vi "XYZ_translation_doubleside.vi"() -> ()   [LabVIEW 2021]
uses:
  C:/Program Files (x86)/Control/SC3U.dll
  Program Files (x86)/Control/SC3U.dll
  <instrlib>/Xbox-One-Controller/Private/Type Defs/Indicators/Controller.ctl
  <instrlib>/Xbox-One-Controller/Private/Type Defs/Indicators/A.ctl
  <instrlib>/Xbox-One-Controller/Private/Type Defs/Indicators/B.ctl
  <instrlib>/Xbox-One-Controller/Private/Type Defs/Indicators/X.ctl
  <instrlib>/Xbox-One-Controller/Private/Type Defs/Indicators/Y.ctl
  <instrlib>/Xbox-One-Controller/Private/Type Defs/Indicators/Left Bumper.ctl
  <instrlib>/Xbox-One-Controller/Private/Type Defs/Indicators/Right Bumper.ctl
  <instrlib>/Xbox-One-Controller/Private/Type Defs/Indicators/View.ctl
  <instrlib>/Xbox-One-Controller/Private/Type Defs/Indicators/Menu.ctl
  <instrlib>/Xbox-One-Controller/Private/Type Defs/Indicators/Thumbstick_Analog.ctl
  <instrlib>/Xbox-One-Controller/Private/Type Defs/Indicators/Slider.ctl
  <instrlib>/Xbox-One-Controller/Private/Type Defs/Indicators/DPad.ctl
  <vilib>/Platform/TimedLoop/XDataNode/timing_clust.ctl
  <vilib>/Platform/TimedLoop/XDataNode/nitl_modes.ctl
  <vilib>/Platform/TimedLoop/XDataNode/wakeup.ctl
  <instrlib>/Xbox-One-Controller/Public/Open First Controller.vi
  <vilib>/Platform/TimedLoop/XDataNode/XDataNode.xnode
  <vilib>/Platform/TimedLoop/XDataNode/XDNodeRunTimeDep.lvlib
  <instrlib>/Xbox-One-Controller/LMH-Xbox-One-Controller.lvlib
panel:
  in  "Front Panel Window:Is Frontmost":bool
  in  "Displace Stamp Y":i64=1
  in  "Displace Stamp X":i64=1
  in  "Displace Sample R":i64=1
  out "Pos Stamp Y":dbl
  out "Pos Stamp X":dbl
  out "Pos Sample R":dbl
  in  "Displace Divided by 5":bool caption="Boolean 2"
  in  "Displace Multip by 5":bool caption="Boolean"
  out "Pos Sample X":dbl
  out "Pos Sample Z":dbl
  in  "Displace Sample Z":i64=1
  out "Pos Sample Y":dbl
  in  "Displace Sample Y":i64
  in  "Stop Button":bool
  out "Controller":T1={"A Button"=FALSE, "B Button"=FALSE, "X Button"=FALSE, "Y Button"=FALSE, "Left Bumper"=FALSE, "Right Bumper"=FALSE, "View Button"=FALSE, "Menu Button"=FALSE, "Left Stick"={[], []}, "Right Stick"={[], []}, "Trigger"=0, "D-Pad"=5} {"Trigger" scale=32767.0..-32768.0}
  in  "SC3U":refnum<k24>(container)
  in  "Com Close":bool
  in  "Displace Sample X":i64
  out "ConnectStatus":bool
  out "ComUsing":i16
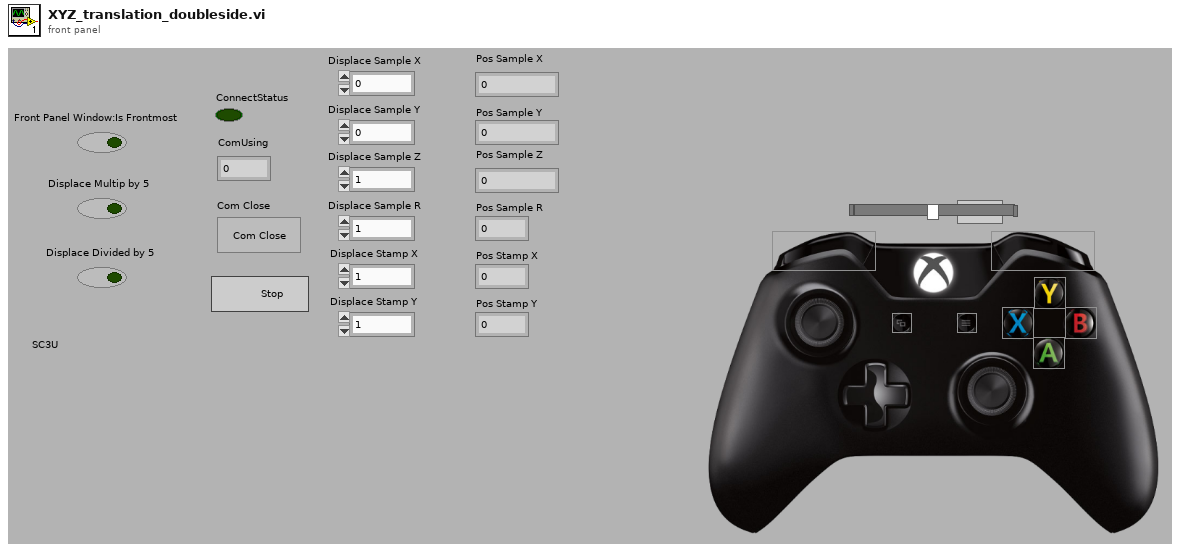
[diagram p1: front panel]
types:
  T1 = typedef "LMH-Xbox-One-Controller.lvlib/Controller.ctl" = cluster{"A Button":T2, "B Button":T3, "X Button":T4, "Y Button":T5, "Left Bumper":T6, "Right Bumper":T7, "View Button":T8, "Menu Button":T9, "Left Stick":T10, "Right Stick":T10, "Trigger":T11, "D-Pad":T12}
  T2 = typedef "LMH-Xbox-One-Controller.lvlib/A.ctl" = bool
  T3 = typedef "LMH-Xbox-One-Controller.lvlib/B.ctl" = bool
  T4 = typedef "LMH-Xbox-One-Controller.lvlib/X.ctl" = bool
  T5 = typedef "LMH-Xbox-One-Controller.lvlib/Y.ctl" = bool
  T6 = typedef "LMH-Xbox-One-Controller.lvlib/Left Bumper.ctl" = bool
  T7 = typedef "LMH-Xbox-One-Controller.lvlib/Right Bumper.ctl" = bool
  T8 = typedef "LMH-Xbox-One-Controller.lvlib/View.ctl" = bool
  T9 = typedef "LMH-Xbox-One-Controller.lvlib/Menu.ctl" = bool
  T10 = typedef "LMH-Xbox-One-Controller.lvlib/Thumbstick_Analog.ctl" = cluster{i32[], i32[]}
  T11 = typedef "LMH-Xbox-One-Controller.lvlib/Slider.ctl" = i32
  T12 = typedef "LMH-Xbox-One-Controller.lvlib/DPad.ctl" = u16
  T13 = typedef "XDNodeRunTimeDep.lvlib/timing_clust.ctl" = cluster{"Expected End [f-1]":u64, "Actual End [f-1]":u64, "Finished Late? [f-1]":bool, "Expected End [i-1]":u64, "Actual End [i-1]":u64, "Finished Late? [i-1]":bool, "Expected Start [i]":u64, "Actual Start [i]":u64, "Expected Start [f]":u64, "Actual Start [f]":u64, "Source Name":string, "Structure Name":string, "Period":i64, "Deadline":i64, "Offset":i64, "Start":i64, "Priority":i32, "Timeout":i32, "Mode":T14, "Wakeup Reason":T15, "Error":errorcluster, "Source Type":string, "Secondary Source Type":string, "Global End Time":u64, "Global Start Time":u64, "Frame Duration":u64, "Iteration Duration":u64, "Assigned CPU":i32, "I/O Scan Engine Mode":u32}
  T14 = typedef "XDNodeRunTimeDep.lvlib/nitl_modes.ctl" = enum32{"No Change", "Process missed periods, maintain original phase", "Discard missed periods, maintain original phase", "Process missed periods, ignore original phase", "Discard missed periods, ignore original phase"}
  T15 = typedef "XDNodeRunTimeDep.lvlib/wakeup.ctl" = enum32{"Normal", "Aborted", "Asynchronous wakeup", "Timing source error", "Timed loop error", "Timeout"}
  T16 = typedef "LMH-Xbox-One-Controller.lvlib/Xbox One Controller Ref.ctl" = cluster{"Controller Ref":refnum<k1>, "Event Refnum":refnum<event-registration>, "Worker Ref":refnum<vi>}
  T17 = typedef "LMH-Xbox-One-Controller.lvlib/All Axis Data.ctl" = cluster{"Left Stick":cluster{"X Axis":i32, "Y Axis":i32}, "Right Stick":cluster{"X Axis":i32, "Y Axis":i32}, "Triggers":i32, "D-Pad":T18}
  T18 = typedef "LMH-Xbox-One-Controller.lvlib/DPad Enum.ctl" = enum16{"Idle", "Up", "Up / Right", "Right", "Down / Right", "Down", "Down / Left", "Left", "Up / Left"}
  T19 = typedef "LMH-Xbox-One-Controller.lvlib/All Buttons Visual.ctl" = cluster{"A":T2, "B":T3, "X":T4, "Y":T5, "Left Bumper":T6, "Right Bumper":T7, "View Button":T8, "Menu Button":T9, "Left Stick":T20, "Right Stick":T20}
  T20 = typedef "LMH-Xbox-One-Controller.lvlib/Thumbstick.ctl" = bool
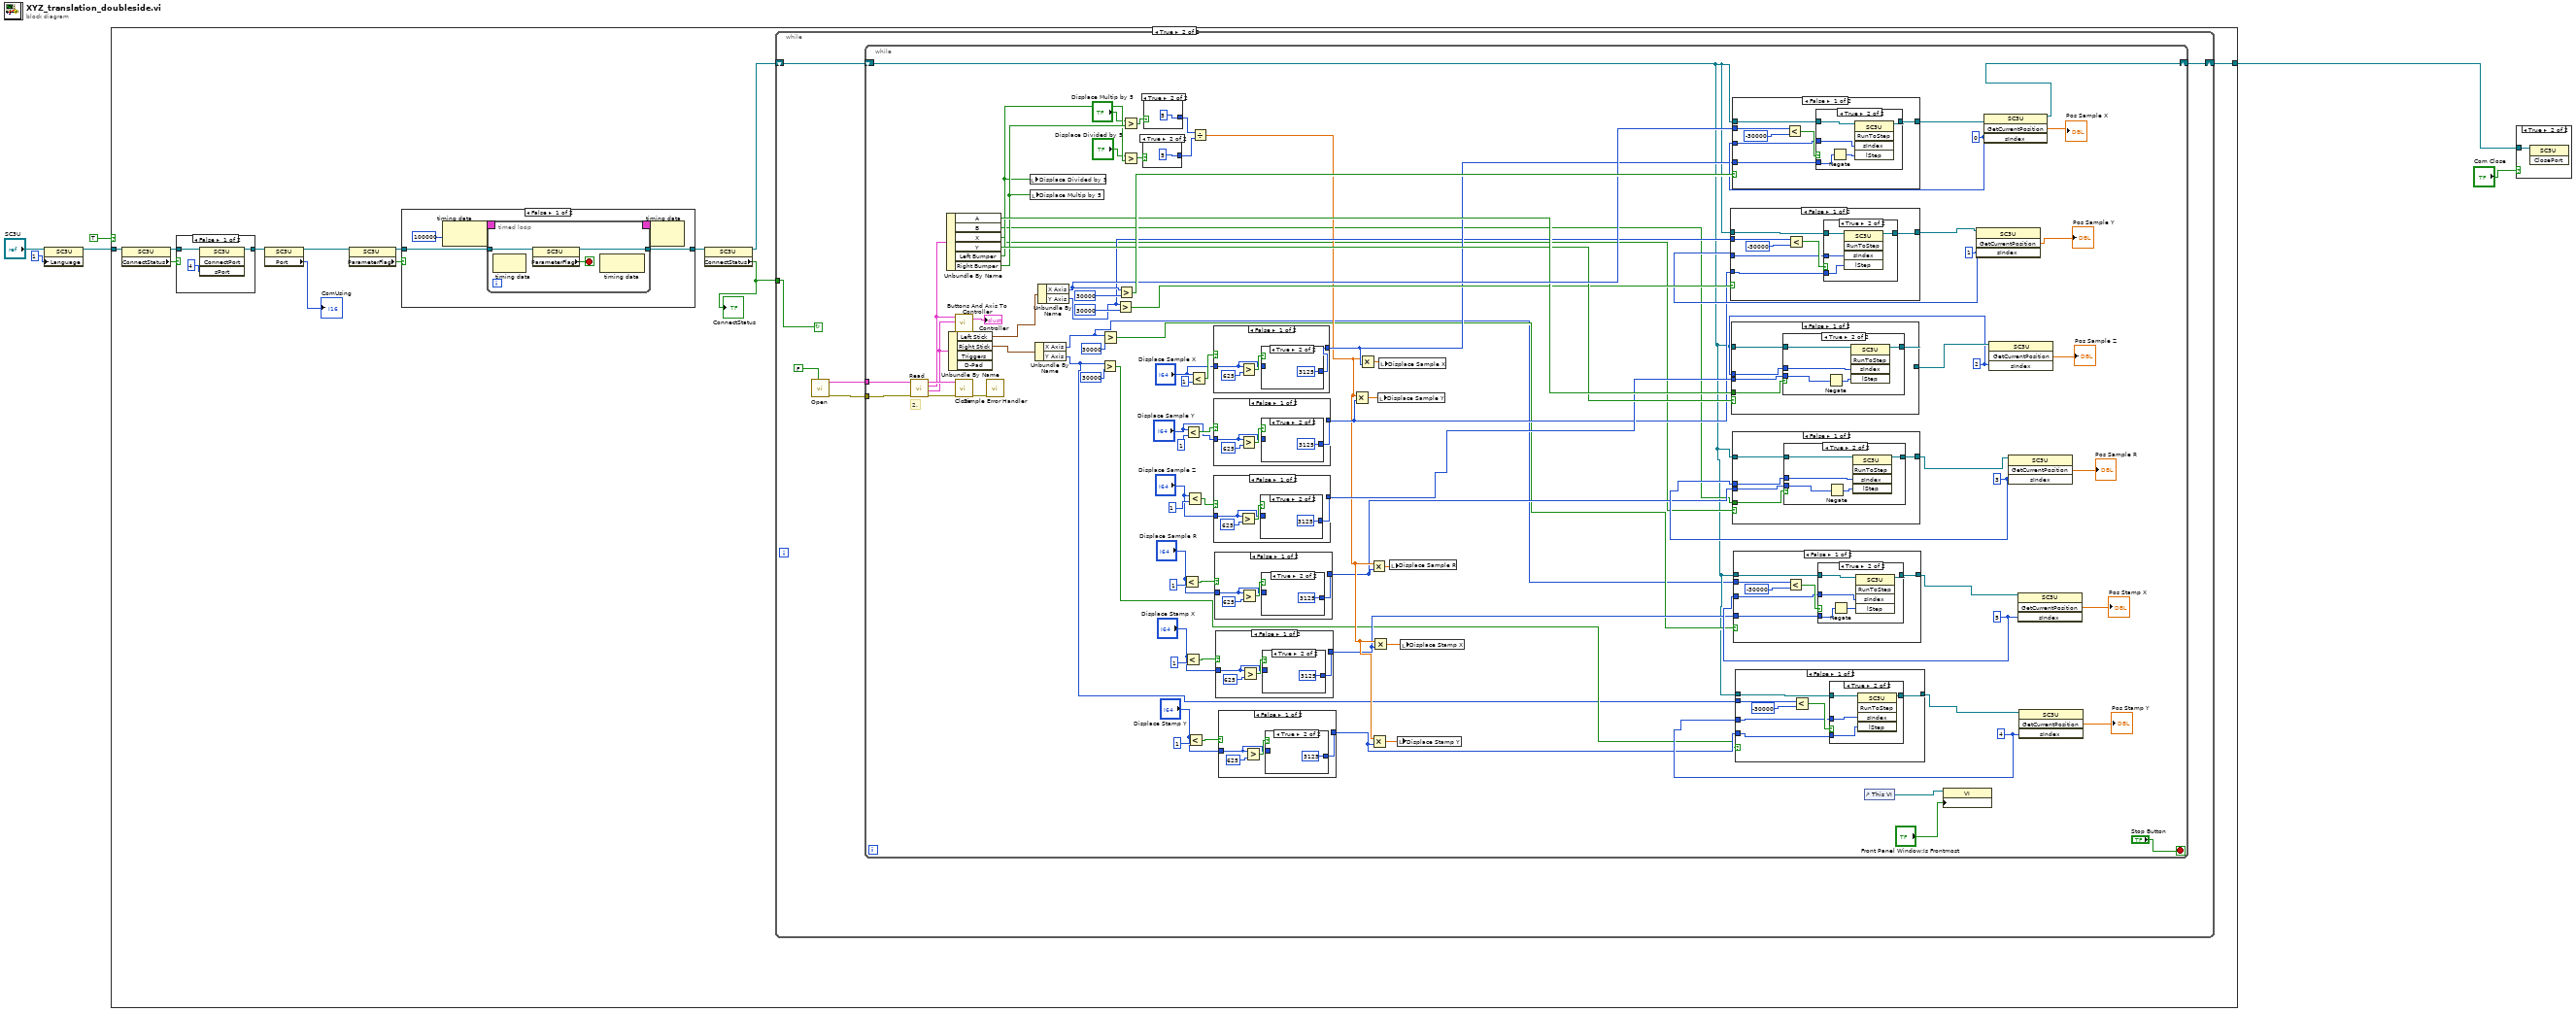
[diagram p0: block diagram]
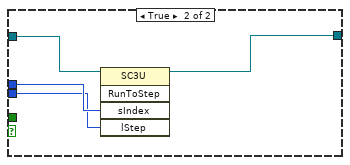
[diagram p5: hidden frame]
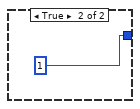
[diagram p7: hidden frame]
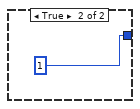
[diagram p9: hidden frame]
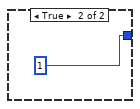
[diagram p11: hidden frame]
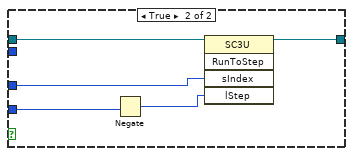
[diagram p13: hidden frame]
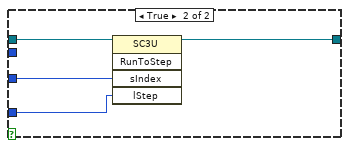
[diagram p15: hidden frame]
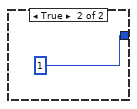
[diagram p17: hidden frame]
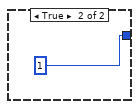
[diagram p19: hidden frame]
diagram:
  n1 = property class="SC3U"(reference="SC3U", "Language"=i16 1 ("intLanguage")) -> (reference out=w1:refnum<k24>)  [unwired: 1 in, 1 out]
  n2 = case shown="True" TRUE {
    tunnel: [_ w8] -> w2
    tunnel: w1 -> [_ w17]
    frame False {
    }
    frame True {
      n3 = property class="SC3U"(reference=w17) -> (reference out=w16:refnum<k24>, "ConnectStatus"=w15:bool)  [unwired: 1 in, 1 out]
      n4 = case shown="False" w15 {
        tunnel: w16 -> [w273 w274]
        tunnel: [w272 w274] -> w14
        frame False {
          n5 = invoke class="SC3U" method="ConnectPort"(reference=w273, "sPort"=i16 4 ("ComUsing")) -> (reference out=w272:refnum<k24>)  [unwired: 2 in, 3 out]
        }
        frame True {
        }
      }
      n6 = property class="SC3U"(reference=w14) -> (reference out=w12:refnum<k24>, "Port"=→"ComUsing":i16)  [unwired: 1 in, 1 out]
      n7 = property class="SC3U"(reference=w12) -> (reference out=w11:refnum<k24>, "ParameterFlag"=w10:bool)  [unwired: 1 in, 1 out]
      n8 = case shown="False" w10 {
        tunnel: w11 -> [w257 w270]
        tunnel: [w256 w270] -> w18
        frame False {
          n9 = node-c288(i64 100000 ("周期")) -> (w260:T13)
          n10 = timed-loop {
            timing: w260 -> [_]
            timing-out: [_] -> w259
            tunnel: w257 -> [w263]
            tunnel: [w262] -> w256
            stop <- w261 stop-if-true
            n11 = node-c288() -> ()  [unwired: 1 in, 1 out]
            n12 = property class="SC3U"(reference=w263) -> (reference out=w262:refnum<k24>, "ParameterFlag"=w261:bool)  [unwired: 1 in, 1 out]
            n13 = node-c288() -> ()  [unwired: 1 in, 1 out]
          }
          n14 = node-c288(w259) -> ()  [unwired: 1 out]
        }
        frame True {
        }
      }
      n15 = property class="SC3U"(reference=w18) -> (reference out=w7:refnum<k24>, "ConnectStatus"=w9:bool)  [unwired: 1 in, 1 out]
      "ConnectStatus" <- w9
      n16 = while {
        shift-right: [w24] -> w8
        shift-left: w7 -> [w23]
        tunnel: w9 -> [w22]
        stop <- w22 continue-if-true
        n17 = call-poly <instrlib>:"Open.vi"("Enable Events (T)"=FALSE) -> ("Error Out"=w21:errorcluster, "Xbox One Controller"=w19:T16)  [unwired: 8 in, 1 out]
        n18 = while {
          tunnel: w19 -> [w109]
          tunnel: w21 -> [w108]
          shift-right: [w39] -> w24
          shift-left: w23 -> [w29]
          stop <- "Stop Button" stop-if-true
          w56 = i16 4 ("sIndex")
          w58 = i16 5 ("sIndex")
          w35 = i16 3 ("sIndex")
          w76 = 2
          w77 = 1
          w78 = 0
          # "2."
          n19 = call <instrlib>:"Read.vi"("Error In"=w108, "Xbox One Controller Ref"=w109) -> ("Error Out"=w106:errorcluster, "All Axis"=w104:T17, "Buttons"=w99:T19, "Xbox One Controller Ref"=w105:T16)  [unwired: 6 in]
          n20 = Unbundle By Name(w99) -> ("A"=w98:T2, "B"=w30:T3, "X"=w31:T4, "Y"=w97:T5, "Left Bumper"=w93:T6, "Right Bumper"=w94:T7)
          n21 = Unbundle By Name(w104) -> ("Left Stick"=w111:cluster{"X Axis":i32, "Y Axis":i32}, "Right Stick"=w95:cluster{"X Axis":i32, "Y Axis":i32})  [unwired: 2 out]
          n22 = call <instrlib>:"Buttons And Axis To Controller.vi"("All Axis"=w104, "Buttons"=w99) -> ("Controller"=→"Controller":T1)  [unwired: 5 in]
          n23 = call <instrlib>:"Close.vi"("Error In"=w106, "Xbox One Controller Ref"=w105) -> ("Error Out"=w107:errorcluster)  [unwired: 9 in]
          n24 = call <vilib>:"Simple Error Handler.vi"("error in (no error)"=w107) -> ()  [unwired: 4 in, 5 out]
          n25 = local write "Displace Divided by 5"(w93) -> ()
          n26 = local write "Displace Multip by 5"(w94) -> ()
          n27 = Unbundle By Name(w95) -> ("X Axis"=w28:i32, "Y Axis"=w27:i32)
          n28 = Unbundle By Name(w111) -> ("X Axis"=w101:i32, "Y Axis"=w46:i32)
          n29 = Greater?(x=w27, y=30000) -> (0:w33:bool)
          n30 = Greater?(x=w28, y=30000) -> (0:w32:bool)
          n31 = Greater?(x=w46, y=30000) -> (0:w92:bool)
          n32 = Greater?(x=w101, y=30000) -> (0:w102:bool)
          n33 = Greater?(x="Displace Multip by 5", y=w94) -> (0:w90:T7)
          n34 = Greater?(x="Displace Divided by 5", y=w93) -> (0:w89:T6)
          n35 = case shown="True" w89 {
            tunnel: [1 5] -> w66
            frame False {
            }
            frame True {
            }
          }
          n36 = case shown="True" w90 {
            tunnel: [1 5] -> w67
            frame False {
            }
            frame True {
            }
          }
          n37 = Less?(x="Displace Sample R", y=i64 1) -> (x < y?=w54:bool)
          n38 = Less?(x="Displace Stamp X", y=i64 1) -> (x < y?=w51:bool)
          n39 = Less?(x="Displace Sample Y", y=i64 1) -> (x < y?=w70:bool)
          n40 = Less?(x="Displace Sample Z", y=i64 1) -> (x < y?=w85:bool)
          n41 = Less?(x="Displace Stamp Y", y=i64 1) -> (x < y?=w48:bool)
          n42 = Less?(x="Displace Sample X", y=i64 1) -> (x < y?=w71:bool)
          n43 = Divide(x=w67, y=w66) -> (x/y=w45:dbl)
          n44 = case shown="False" w71 {
            tunnel: "Displace Sample X" -> [w182 _]
            tunnel: [w183 1] -> w63
            frame False {
              n45 = Greater?(x=w182, y=i64 625) -> (0:w184:bool)
              n46 = case shown="True" w184 {
                tunnel: [w186 3125] -> w183
                tunnel: w182 -> [w186 _]
                frame False {
                }
                frame True {
                }
              }
            }
            frame True {
            }
          }
          n47 = case shown="False" w70 {
            tunnel: "Displace Sample Y" -> [w189 _]
            tunnel: [w190 1] -> w64
            frame False {
              n48 = Greater?(x=w189, y=i64 625) -> (0:w191:bool)
              n49 = case shown="True" w191 {
                tunnel: [w193 3125] -> w190
                tunnel: w189 -> [w193 _]
                frame False {
                }
                frame True {
                }
              }
            }
            frame True {
            }
          }
          n50 = case shown="False" w85 {
            tunnel: "Displace Sample Z" -> [w245 _]
            tunnel: [w246 1] -> w74
            frame False {
              n51 = Greater?(x=w245, y=i64 625) -> (0:w247:bool)
              n52 = case shown="True" w247 {
                tunnel: [w249 3125] -> w246
                tunnel: w245 -> [w249 _]
                frame False {
                }
                frame True {
                }
              }
            }
            frame True {
            }
          }
          n53 = case shown="False" w54 {
            tunnel: "Displace Sample R" -> [w141 _]
            tunnel: [w142 1] -> w34
            frame False {
              n54 = Greater?(x=w141, y=i64 625) -> (0:w143:bool)
              n55 = case shown="True" w143 {
                tunnel: [w145 3125] -> w142
                tunnel: w141 -> [w145 _]
                frame False {
                }
                frame True {
                }
              }
            }
            frame True {
            }
          }
          n56 = case shown="False" w51 {
            tunnel: "Displace Stamp X" -> [w134 _]
            tunnel: [w135 1] -> w41
            frame False {
              n57 = Greater?(x=w134, y=i64 625) -> (0:w136:bool)
              n58 = case shown="True" w136 {
                tunnel: [w138 3125] -> w135
                tunnel: w134 -> [w138 _]
                frame False {
                }
                frame True {
                }
              }
            }
            frame True {
            }
          }
          n59 = case shown="False" w48 {
            tunnel: "Displace Stamp Y" -> [w127 _]
            tunnel: [w128 1] -> w40
            frame False {
              n60 = Greater?(x=w127, y=i64 625) -> (0:w129:bool)
              n61 = case shown="True" w129 {
                tunnel: [w131 3125] -> w128
                tunnel: w127 -> [w131 _]
                frame False {
                }
                frame True {
                }
              }
            }
            frame True {
            }
          }
          n62 = Multiply(x=w45, y=w64) -> (x*y=w65:dbl)
          n63 = Multiply(x=w45, y=w63) -> (x*y=w87:dbl)
          n64 = Multiply(x=w45, y=w34) -> (x*y=w42:dbl)
          n65 = Multiply(x=w45, y=w40) -> (x*y=w43:dbl)
          n66 = Multiply(x=w45, y=w41) -> (x*y=w44:dbl)
          n67 = local write "Displace Sample Y"(w65) -> ()
          n68 = local write "Displace Sample X"(w87) -> ()
          n69 = local write "Displace Sample R"(w42) -> ()
          n70 = local write "Displace Stamp Y"(w43) -> ()
          n71 = local write "Displace Stamp X"(w44) -> ()
          n72 = case shown="False" w92 {
            tunnel: [w216 w225] -> w79
            tunnel: w29 -> [w217 w227]
            tunnel: w46 -> [w215 _]
            tunnel: w77 -> [w212 w226]
            tunnel: w64 -> [w211 w223]
            frame False {
              n73 = Less?(x=w215, y=-30000) -> (x < y?=w213:bool)
              n74 = case shown="True" w213 {
                tunnel: w217 -> [w218 w222]
                tunnel: [w218 w220] -> w216
                tunnel: w212 -> [_ w221]
                tunnel: w211 -> [_ w219]
                frame False {
                }
                frame True {
                  n75 = invoke class="SC3U" method="RunToStep"(reference=w222, "sIndex"=w221, "lStep"=w219) -> (reference out=w220:refnum<k24>)  [unwired: 2 in, 4 out]
                }
              }
            }
            frame True {
              n76 = Negate(x=w223) -> (-x=w224:i64)
              n77 = invoke class="SC3U" method="RunToStep"(reference=w227, "sIndex"=w226, "lStep"=w224) -> (reference out=w225:refnum<k24>)  [unwired: 2 in, 4 out]
            }
          }
          n78 = case shown="False" w97 {
            tunnel: w76 -> [w198 w210]
            tunnel: w74 -> [w197 w209]
            tunnel: w29 -> [w200 w208]
            tunnel: [w199 w207] -> w82
            tunnel: w98 -> [w196 _]
            frame False {
              n79 = case shown="True" w196 {
                tunnel: w200 -> [w201 w206]
                tunnel: [w201 w205] -> w199
                tunnel: w198 -> [_ w204]
                tunnel: w197 -> [_ w202]
                frame False {
                }
                frame True {
                  n80 = Negate(x=w202) -> (-x=w203:i64)
                  n81 = invoke class="SC3U" method="RunToStep"(reference=w206, "sIndex"=w204, "lStep"=w203) -> (reference out=w205:refnum<k24>)  [unwired: 2 in, 4 out]
                }
              }
            }
            frame True {
              n82 = invoke class="SC3U" method="RunToStep"(reference=w208, "sIndex"=w210, "lStep"=w209) -> (reference out=w207:refnum<k24>)  [unwired: 2 in, 4 out]
            }
          }
          n83 = case shown="False" w102 {
            tunnel: [w233 w242] -> w84
            tunnel: w29 -> [w234 w244]
            tunnel: w101 -> [w232 _]
            tunnel: w78 -> [w229 w243]
            tunnel: w63 -> [w228 w241]
            frame False {
              n84 = Less?(x=w232, y=-30000) -> (x < y?=w230:bool)
              n85 = case shown="True" w230 {
                tunnel: w234 -> [w235 w240]
                tunnel: [w235 w237] -> w233
                tunnel: w229 -> [_ w238]
                tunnel: w228 -> [_ w236]
                frame False {
                }
                frame True {
                  n86 = Negate(x=w236) -> (-x=w239:i64)
                  n87 = invoke class="SC3U" method="RunToStep"(reference=w240, "sIndex"=w238, "lStep"=w239) -> (reference out=w237:refnum<k24>)  [unwired: 2 in, 4 out]
                }
              }
            }
            frame True {
              n88 = invoke class="SC3U" method="RunToStep"(reference=w244, "sIndex"=w243, "lStep"=w241) -> (reference out=w242:refnum<k24>)  [unwired: 2 in, 4 out]
            }
          }
          n89 = case shown="False" w31 {
            tunnel: w35 -> [w114 w126]
            tunnel: w34 -> [w113 w125]
            tunnel: w29 -> [w116 w124]
            tunnel: [w115 w123] -> w36
            tunnel: w30 -> [w112 _]
            frame False {
              n90 = case shown="True" w112 {
                tunnel: w116 -> [w117 w122]
                tunnel: [w117 w121] -> w115
                tunnel: w114 -> [_ w120]
                tunnel: w113 -> [_ w118]
                frame False {
                }
                frame True {
                  n91 = Negate(x=w118) -> (-x=w119:i64)
                  n92 = invoke class="SC3U" method="RunToStep"(reference=w122, "sIndex"=w120, "lStep"=w119) -> (reference out=w121:refnum<k24>)  [unwired: 2 in, 4 out]
                }
              }
            }
            frame True {
              n93 = invoke class="SC3U" method="RunToStep"(reference=w124, "sIndex"=w126, "lStep"=w125) -> (reference out=w123:refnum<k24>)  [unwired: 2 in, 4 out]
            }
          }
          n94 = case shown="False" w32 {
            tunnel: [w170 w179] -> w59
            tunnel: w29 -> [w171 w181]
            tunnel: w28 -> [w169 _]
            tunnel: w58 -> [w166 w180]
            tunnel: w41 -> [w165 w178]
            frame False {
              n95 = Less?(x=w169, y=-30000) -> (x < y?=w167:bool)
              n96 = case shown="True" w167 {
                tunnel: w171 -> [w172 w177]
                tunnel: [w172 w174] -> w170
                tunnel: w166 -> [_ w175]
                tunnel: w165 -> [_ w173]
                frame False {
                }
                frame True {
                  n97 = Negate(x=w173) -> (-x=w176:i64)
                  n98 = invoke class="SC3U" method="RunToStep"(reference=w177, "sIndex"=w175, "lStep"=w176) -> (reference out=w174:refnum<k24>)  [unwired: 2 in, 4 out]
                }
              }
            }
            frame True {
              n99 = invoke class="SC3U" method="RunToStep"(reference=w181, "sIndex"=w180, "lStep"=w178) -> (reference out=w179:refnum<k24>)  [unwired: 2 in, 4 out]
            }
          }
          n100 = case shown="False" w33 {
            tunnel: [w153 w162] -> w57
            tunnel: w29 -> [w154 w164]
            tunnel: w27 -> [w152 _]
            tunnel: w56 -> [w149 w163]
            tunnel: w40 -> [w148 w161]
            frame False {
              n101 = Less?(x=w152, y=-30000) -> (x < y?=w150:bool)
              n102 = case shown="True" w150 {
                tunnel: w154 -> [w155 w159]
                tunnel: [w155 w157] -> w153
                tunnel: w149 -> [_ w158]
                tunnel: w148 -> [_ w156]
                frame False {
                }
                frame True {
                  n103 = invoke class="SC3U" method="RunToStep"(reference=w159, "sIndex"=w158, "lStep"=w156) -> (reference out=w157:refnum<k24>)  [unwired: 2 in, 4 out]
                }
              }
            }
            frame True {
              n104 = Negate(x=w161) -> (-x=w160:i64)
              n105 = invoke class="SC3U" method="RunToStep"(reference=w164, "sIndex"=w163, "lStep"=w160) -> (reference out=w162:refnum<k24>)  [unwired: 2 in, 4 out]
            }
          }
          n106 = control-ref of="This VI"() -> (w26:refnum<vi>)
          n107 = property class="VI"(reference=w26, "Front Panel.IsFrontmost"="Front Panel Window:Is Frontmost") -> ()  [unwired: 1 in, 2 out]
          n108 = invoke class="SC3U" method="GetCurrentPosition"(reference=w79, "sIndex"=w77) -> ("GetCurrentPosition"=→"Pos Sample Y":dbl)  [unwired: 2 in, 3 out]
          n109 = invoke class="SC3U" method="GetCurrentPosition"(reference=w84, "sIndex"=w78) -> (reference out=w39:refnum<k24>, "GetCurrentPosition"=→"Pos Sample X":dbl)  [unwired: 2 in, 2 out]
          n110 = invoke class="SC3U" method="GetCurrentPosition"(reference=w82, "sIndex"=w76) -> ("GetCurrentPosition"=→"Pos Sample Z":dbl)  [unwired: 2 in, 3 out]
          n111 = invoke class="SC3U" method="GetCurrentPosition"(reference=w36, "sIndex"=w35) -> ("GetCurrentPosition"=→"Pos Sample R":dbl)  [unwired: 2 in, 3 out]
          n112 = invoke class="SC3U" method="GetCurrentPosition"(reference=w59, "sIndex"=w58) -> ("GetCurrentPosition"=→"Pos Stamp X":dbl)  [unwired: 2 in, 3 out]
          n113 = invoke class="SC3U" method="GetCurrentPosition"(reference=w57, "sIndex"=w56) -> ("GetCurrentPosition"=→"Pos Stamp Y":dbl)  [unwired: 2 in, 3 out]
        }
      }
    }
  }
  n114 = case shown="True" "Com Close" {
    tunnel: w2 -> [_ w275]
    frame False {
    }
    frame True {
      n115 = invoke class="SC3U" method="ClosePort"(reference=w275) -> ()  [unwired: 2 in, 3 out]
    }
  }
